vi "Switch Valve.vi"(8 "Error In":errorcluster, 9 "Open (F:close)":bool, 10 "Channel (-1:Main)":i32=-1, 11 "VISA resource name":refnum<visa-resource-name>) -> (0 "Error Out":errorcluster, 3 "dup VISA resource name":refnum<visa-resource-name>)   [LabVIEW 2011, in "MGC647C.lvlib"]
doc: "Switch valve of a channel."
uses:
  <instrlib>/MGC647C/MGC647C.lvlib
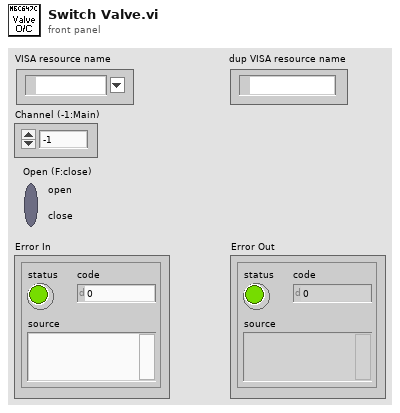
[diagram p1: front panel]
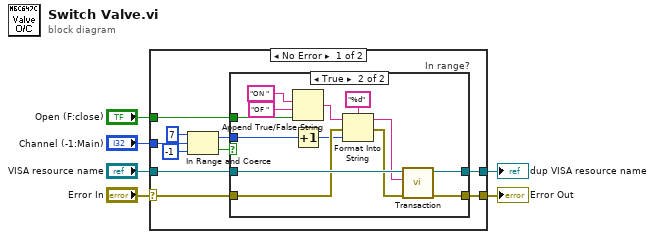
[diagram p0: block diagram]
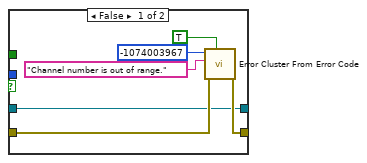
[diagram p2: hidden frame]
diagram:
  n1 = case shown="No Error" "Error In" {
    selector: "Error In" -> [w13 w37]
    tunnel: "VISA resource name" -> [w16 w36]
    tunnel: [w15 w36] -> w5
    tunnel: [w14 w37] -> w4
    tunnel: "Channel (-1:Main)" -> [w10 _]
    tunnel: "Open (F:close)" -> [w7 _]
    frame No Error {
      n2 = In Range and Coerce(upper limit=7, x=w10, lower limit=-1) -> (coerced(x)=w9:i32, In Range?=w8:bool)
      n3 = case "In range?" shown="True" w8 {
        tunnel: w16 -> [w20 w35]
        tunnel: [w20 w34] -> w15
        tunnel: [w21 w27] -> w14
        tunnel: w13 -> [w22 w33]
        tunnel: w9 -> [_ w31]
        tunnel: w7 -> [_ w25]
        frame False {
          n4 = call <vilib>:"Error Cluster From Error Code.vi"("show call chain? (False)"=TRUE, "error in (no error)"=w22, "error message (\"\")"="Channel number is out of range." ("error message (\"\")"), "error code (0)"=-1074003967) -> ("error out"=w21:errorcluster)  [unwired: 5 in]
        }
        frame True {
          n5 = Append True/False String(1:w25, 2:"OF " ("string (\"\")"), 3:"ON " ("string (\"\")")) -> (0:w26:string)  [unwired: 1 in]
          n6 = Increment(x=w31) -> (x+1=w30:i32)
          n7 = Format Into String(format string="%d", initial string=w26, error in=w33, w30) -> (resulting string=w29:string, error out=w32:errorcluster)
          n8 = call <instrlib>:"Transaction.vi"("Error In"=w32, "Command"=w29, "VISA resource name"=w35) -> ("Error Out"=w27:errorcluster, "dup VISA resource name"=w34:refnum<visa-resource-name>)  [unwired: 6 in, 1 out]
        }
      }
    }
    frame Error {
    }
  }
  "dup VISA resource name" <- w5
  "Error Out" <- w4
